vi "Synchronised one pulse signal generation and acquisition.vi"() -> ()   [LabVIEW 2010]
doc: "This example shows how to acquire 16k samples of signal on fast analog inputs. Signal will be acquired simultaneously with generated signal. Time length of the acquired signal depends on the time scale of a buffer that can be set with a decimation factor. Decimations and time scales of a buffer are given in the table below. Voltage range of fast analog inputs on the Red Pitaya depends on gain setting that can be set by jumpers. HV setting is for input range to ±20V, while LV sets input range to ±1V."
uses:
  RedPitaya.lvlib
panel:
  in  "Number of repeated Bursts":i32=-1 min=-1 max=50000
  in  "Number of generated Signals / Burst":i32=1 min=-1 max=50000
  in  "Trigger Level (0 V)":dbl=0.5 min=-20.0 max=20.1
  in  "Delay (# Samples)":i32
  in  "Averaging":enum16{"None", "AVG ON", "AVG OFF"}(ring)
  in  "Decimation":u32(ring)=1 items=["65536"=65536, "8192"=8192, "1024"=1024, "64"=64, "8"=8, "1"=1]
  in  "Total Time of One Burst":i32=-1
  in  "Duty Cycle":i32=-1 min=-1 max=100
  in  "Phase":i32=361
  in  "DC Offset":dbl=2.0
  in  "Frequency (1000 Hz)":i32=50000
  in  "Amplitude(1V)":dbl=1.0
  in  "Waveform Function":u16(ring)=1 items=["", "Sine", "Square", "Triangle", "Sawtooth UP", "Sawtooth Down", "PWM"]
  in  "Channel (1|2)":u16(ring)=1 items=["Channel 1"=1, "Channel 2"=2]
  in  "IP address":string="192.168.178.107"
  out "Waveform Graph":dbl[](graph)
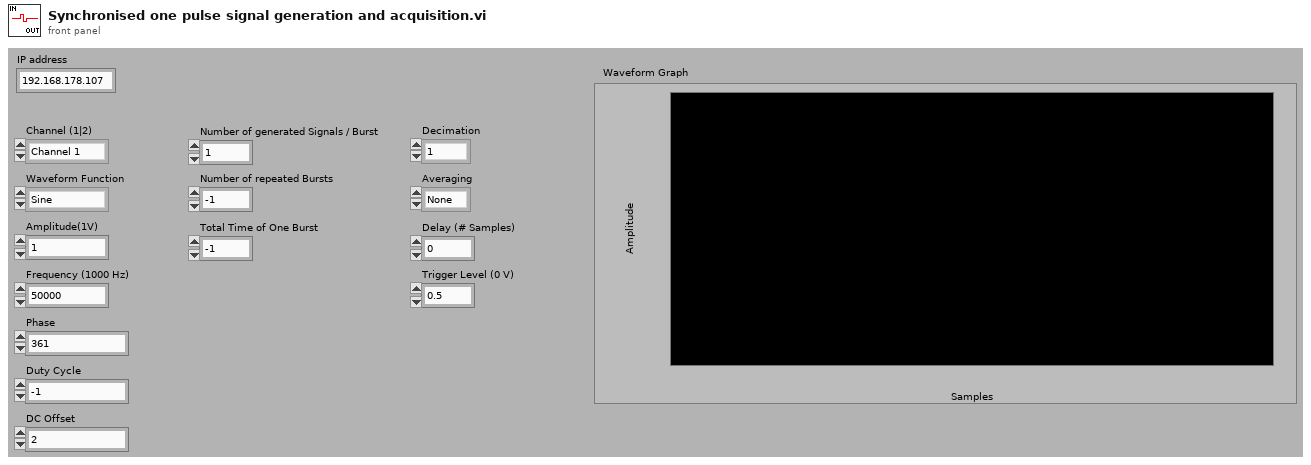
[diagram p1: front panel]
types:
  T1 = enum16{"Disabled", "Now", "Ch1 positive edge", "Ch1 negative edge", "Ch2 positive edge", "Ch2 negative edge", "external positive ege", "external negative edge", "AWG positive edge", "AWG negative edge"}
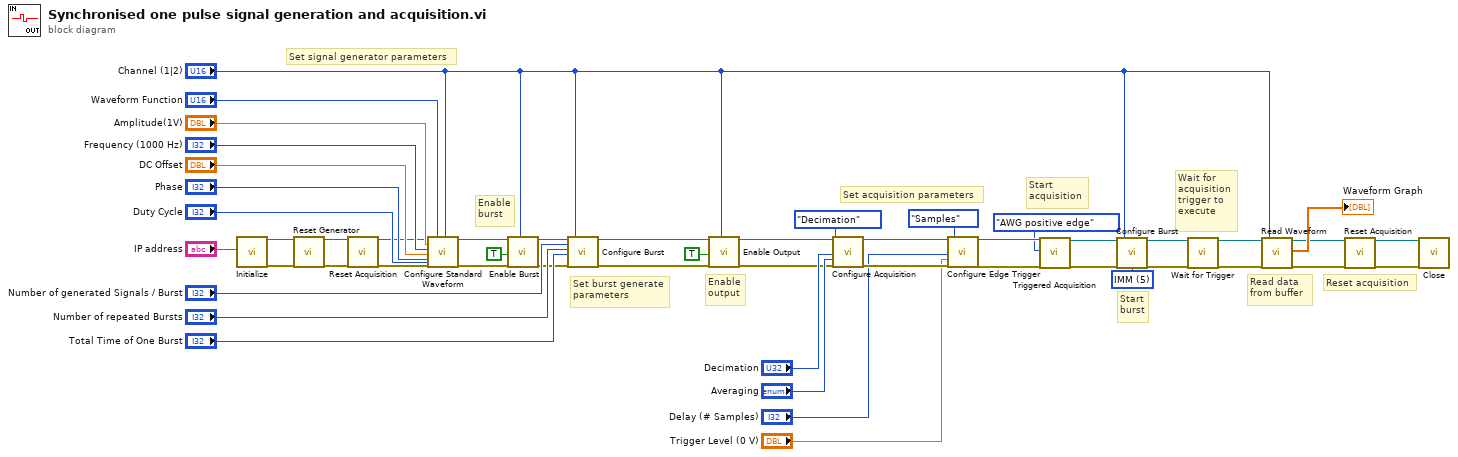
[diagram p0: block diagram]
diagram:
  w35 = u16 5 items=["", "EXT_PE", "EXT_NE", "INT", "GATED", "IMM"] ("Trigger Source")
  # "Reset acquisition"
  # "Read data\nfrom buffer"
  # "Wait for\nacquisition\ntrigger to \nexecute"
  # "Start\nburst"
  # "Start\nacquisition"
  # "Set acquisition parameters"
  # "Enable\nburst"
  # "Enable\noutput"
  # "Set burst generate\nparameters"
  # "Set signal generator parameters"
  n1 = call "Initialize.vi"("IP address"="IP address") -> ("RedPitaya connection out"=w6:refnum<k5>, "error out"=w5:errorcluster)  [unwired: 17 in]
  n2 = call "Reset Generator.vi"("RedPitaya connection in"=w6, "error in"=w5) -> ("RedPitaya connection out"=w4:refnum<k5>, "error out"=w2:errorcluster)  [unwired: 16 in]
  n3 = call "Reset Acquisition.vi"("RedPitaya connection in"=w4, "error in"=w2) -> ("RedPitaya connection out"=w3:refnum<k5>, "error out"=w1:errorcluster)  [unwired: 16 in]
  n4 = call "Configure Standard Waveform.vi"("RedPitaya connection in"=w3, "Amplitude (V)"="Amplitude(1V)", "Frequency"="Frequency (1000 Hz)", "DC Offset"="DC Offset", "Phase"="Phase", "error in"=w1, "Channel #"="Channel (1|2)", "Duty Cycle"="Duty Cycle", "Waveform Function"="Waveform Function") -> ("RedPitaya connection out"=w8:refnum<k5>, "error out"=w7:errorcluster)  [unwired: 9 in]
  n5 = call "Enable Burst.vi"("RedPitaya connection in"=w8, "Generation (T: Enable)"=TRUE, "error in"=w7, "Channel #"="Channel (1|2)") -> ("RedPitaya connection out"=w14:refnum<k5>, "error out"=w9:errorcluster)  [unwired: 14 in]
  n6 = call "Configure Burst.vi"("RedPitaya connection in"=w14, "Number of generated Signals / Burst"="Number of generated Signals / Burst", "Number of repeated Bursts"="Number of repeated Bursts", "Total time of One Burst"="Total Time of One Burst", "error in"=w9, "Channel #"="Channel (1|2)") -> ("RedPitaya connection out"=w44:refnum<k5>, "error out"=w43:errorcluster)  [unwired: 12 in]
  n7 = call "Enable Output.vi"("RedPitaya connection in"=w44, "Generation (T: Enable)"=TRUE, "error in"=w43, "Channel #"="Channel (1|2)") -> ("RedPitaya connection out"=w11:refnum<k5>, "error out"=w10:errorcluster)  [unwired: 14 in]
  n8 = call "Configure Acquisition.vi"("RedPitaya connection in"=w11, "Decimation/Sampling Rate"=enum16{"", "Sampling rate", "Decimation"}."Decimation", "Decimation"="Decimation", "Averaging"="Averaging", "error in"=w10) -> ("RedPitaya connection out"=w46:refnum<k5>, "error out"=w45:errorcluster)  [unwired: 13 in]
  n9 = call "Configure Edge Trigger.vi"("RedPitaya connection in"=w46, "Trigger Delay mode"=enum16{"", "Samples", "Nanoseconds"}."Samples", "Delay (# Samples)"="Delay (# Samples)", "Trigger Level (0 V)"="Trigger Level (0 V)", "error in"=w45) -> ("RedPitaya connection out"=w49:refnum<k5>, "error out"=w48:errorcluster)  [unwired: 13 in]
  n10 = call "Triggered Acquisition.vi"("RedPitaya TCP connection in"=w49, "Trigger Mode"=T1."AWG positive edge", "error in"=w48) -> ("RedPitaya TCP connection out"=w39:refnum<k5>, "error out"=w38:errorcluster)  [unwired: 15 in]
  n11 = call "Configure Burst.vi"("RedPitaya connection in"=w39, "Trigger Source"=w35, "error in"=w38, "Channel #"="Channel (1|2)") -> ("RedPitaya connection out"=w37:refnum<k5>, "error out"=w36:errorcluster)  [unwired: 14 in]
  n12 = call "Wait for Trigger.vi"("RedPitaya TCP connection in"=w37, "error in"=w36) -> ("RedPitaya TCP connection out"=w41:refnum<k5>, "error out"=w40:errorcluster)  [unwired: 16 in]
  n13 = call "Read Waveform.vi"("RedPitaya TCP Connection in"=w41, "error in"=w40, "Channel #"="Channel (1|2)") -> ("RedPitaya TCP Connection out"=w34:refnum<k5>, "Measurement Array"=→"Waveform Graph":dbl[], "error out"=w31:errorcluster)  [unwired: 14 in]
  n14 = call "Reset Acquisition.vi"("RedPitaya connection in"=w34, "error in"=w31) -> ("RedPitaya connection out"=w33:refnum<k5>, "error out"=w32:errorcluster)  [unwired: 16 in]
  n15 = call "Close.vi"("RedPitaya connection in"=w33, "error in"=w32) -> ()  [unwired: 17 in, 1 out]
